vi "control_lasers_and_SMs_TIMING_TRUNCATED_LOOP.vi"() -> ()   [LabVIEW 2021]
uses:
  <vilib>/DAQmx/write.llb/DAQmx Write (Analog 1D DBL NChan 1Samp).vi
  <vilib>/DAQmx/create/channels.llb/DAQmx Create Channel (AO-Voltage-Basic).vi
  <vilib>/DAQmx/miscellaneous.llb/DAQmx Fill In Error Info.vi
panel:
  in  "Y2 (-10-10V)":dbl
  in  "X2 (-10-10V)":dbl
  in  "Continue Cycle?":bool
  out "Full Cycles":i32
  out "Phase I Iterations":i32
  in  "Phase I Duration (sec)":dbl=10.0 format="%.2f"
  in  "Y1 (-10-10V)":dbl
  in  "X1 (-10-10V)":dbl
  in  "Blanking (0-10v)":dbl=10.0
  in  "561 (0-10v)":dbl
  in  "514 (0-10v)":dbl
  in  "488 (0-10v)":dbl
  in  "445 (0-10v)":dbl
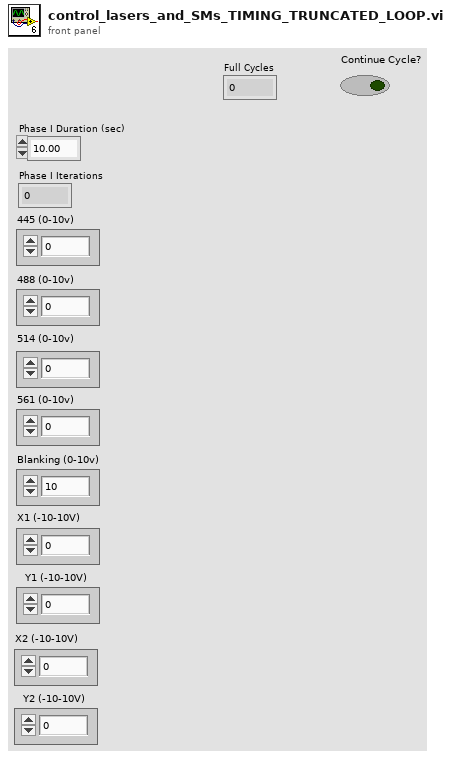
[diagram p1: front panel]
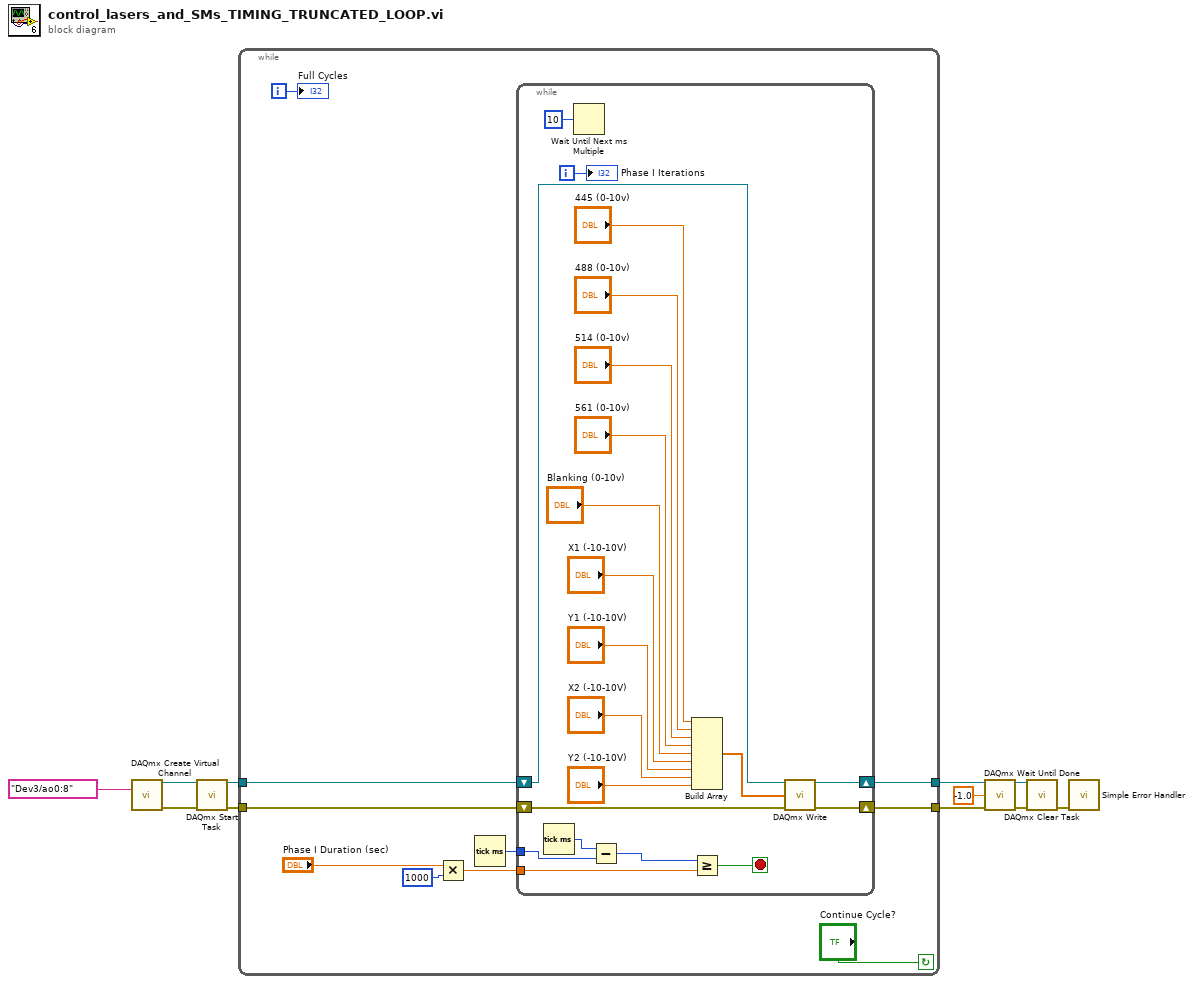
[diagram p0: block diagram]
diagram:
  n1 = call-poly <vilib>:"DAQmx Create Virtual Channel.vi"("physical channels"=tag "Dev3/ao0:8") -> ("task out"=w4:refnum<k21>, "error out"=w3:errorcluster)  [unwired: 13 in]
  n2 = call <vilib>:"DAQmx Start Task.vi"("task/channels in"=w4, "error in"=w3) -> ("task out"=w2:refnum<k21>, "error out"=w1:errorcluster)  [unwired: 12 in]
  n3 = while {
    tunnel: [w13] -> w7
    tunnel: [w12] -> w6
    tunnel: w2 -> [w16]
    tunnel: w1 -> [w15]
    i -> [w17]
    stop <- "Continue Cycle?" continue-if-true
    n4 = Multiply(x="Phase I Duration (sec)", y=1000) -> (x*y=w19:dbl)
    n5 = Tick Count (ms)() -> (millisecond timer value=w20:u32)
    n6 = while {
      shift-right: [w40] -> w13
      shift-left: w16 -> [w42]
      shift-right: [w39] -> w12
      shift-left: w15 -> [w41]
      tunnel: w20 -> [w29]
      tunnel: w19 -> [w25]
      i -> [w30]
      stop <- w26 stop-if-true
      n7 = Tick Count (ms)() -> (millisecond timer value=w28:u32)
      n8 = Wait Until Next ms Multiple(millisecond multiple=10) -> ()  [unwired: 1 out]
      n9 = Subtract(x=w28, y=w29) -> (x-y=w27:u32)
      n10 = Build Array("445 (0-10v)", "488 (0-10v)", "514 (0-10v)", "561 (0-10v)", "Blanking (0-10v)", "X1 (-10-10V)", "Y1 (-10-10V)", "X2 (-10-10V)", "Y2 (-10-10V)") -> (w38:dbl[])
      n11 = Greater Or Equal?(x=w27, y=w25) -> (x >= y?=w26:bool)
      n12 = call-poly <vilib>:"DAQmx Write.vi"("task/channels in"=w42, "data"=w38, "error in"=w41) -> ("task out"=w40:refnum<k21>, "error out"=w39:errorcluster)  [unwired: 10 in, 1 out]
      "Phase I Iterations" <- w30
    }
    "Full Cycles" <- w17
  }
  n13 = call <vilib>:"DAQmx Wait Until Done.vi"("task/channels in"=w7, "timeout (sec)"=-1.0, "error in"=w6) -> ("task out"=w10:refnum<k21>, "error out"=w9:errorcluster)  [unwired: 11 in]
  n14 = call <vilib>:"DAQmx Clear Task.vi"("task in"=w10, "error in"=w9) -> ("error out"=w11:errorcluster)  [unwired: 13 in]
  n15 = call <vilib>:"Simple Error Handler.vi"("error in (no error)"=w11) -> ()  [unwired: 4 in, 5 out]
